vi "buoyfindfirstwp.vi"(0 "X of boat":dbl, 1 "Y of boat":dbl, 2 "Buoy Location Input":T1) -> (3 "X of new waypoint":i32, 4 "Y of new waypoint":i32, 5 "X of Buoy":i32, 6 "Y of Buoy":i32)   [LabVIEW 2014]
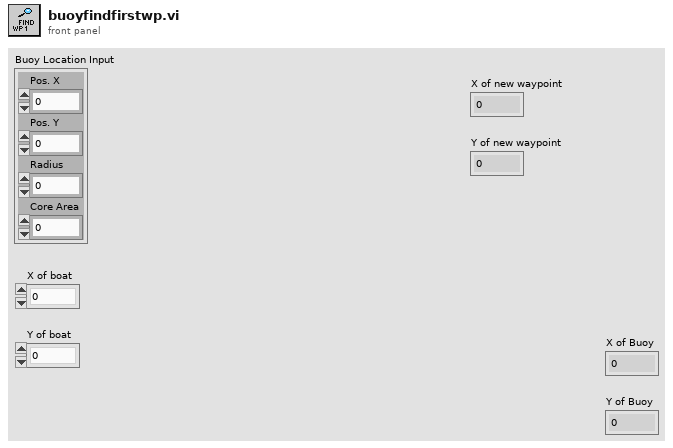
[diagram p1: front panel]
types:
  T1 = cluster{"Pos. X":i32, "Pos. Y":i32, "Radius":i32, "Core Area":i32}
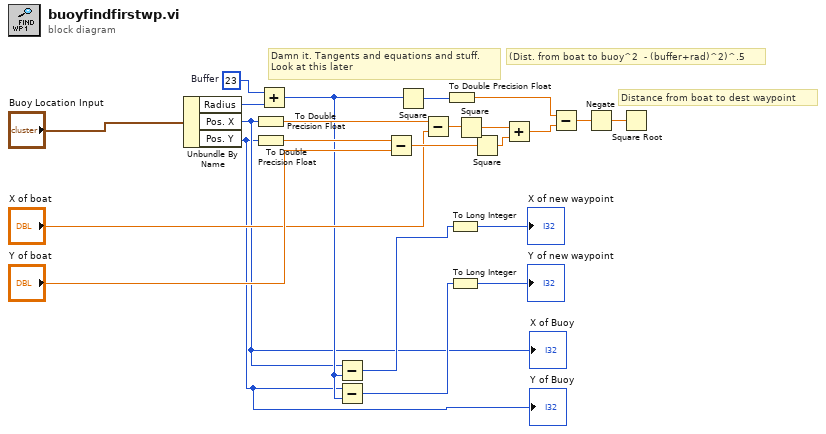
[diagram p0: block diagram]
diagram:
  w21 = 23  # Buffer
  # "Damn it. Tangents and equations and stuff.\nLook at this later"
  # "Distance from boat to dest waypoint"
  # "(Dist. from boat to buoy^2  - (buffer+rad)^2)^.5"
  n1 = Unbundle By Name("Buoy Location Input") -> ("Radius"=w22:i32, "Pos. X"=w2:i32, "Pos. Y"=w1:i32)
  "X of Buoy" <- w2
  "Y of Buoy" <- w1
  n2 = To Double Precision Float(number=w2) -> (double precision float=w11:dbl)
  n3 = To Double Precision Float(number=w1) -> (double precision float=w16:dbl)
  n4 = Add(x=w21, y=w22) -> (x+y=w5:i32)
  n5 = Subtract(x=w2, y=w5) -> (x-y=w4:i32)
  n6 = Subtract(x=w1, y=w5) -> (x-y=w3:i32)
  n7 = Subtract(x=w16, y="Y of boat") -> (x-y=w19:dbl)
  n8 = Square(x=w5) -> (x^2=w9:i32)
  n9 = Subtract(x=w11, y="X of boat") -> (x-y=w20:dbl)
  n10 = To Double Precision Float(number=w9) -> (double precision float=w8:dbl)
  n11 = To Long Integer(number=w4) -> (32bit integer=→"X of new waypoint":i32)
  n12 = To Long Integer(number=w3) -> (32bit integer=→"Y of new waypoint":i32)
  n13 = Square(x=w20) -> (x^2=w17:dbl)
  n14 = Square(x=w19) -> (x^2=w18:dbl)
  n15 = Add(x=w17, y=w18) -> (x+y=w10:dbl)
  n16 = Subtract(x=w8, y=w10) -> (x-y=w7:dbl)
  n17 = Negate(x=w7) -> (-x=w6:dbl)
  n18 = Square Root(x=w6) -> ()  [unwired: 1 out]
